vi "closeMightex.vi"   [LabVIEW 2016]
uses:
  lib/SSClassic_USBCamera_SDK.dll
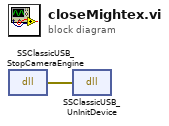
[diagram p0: block diagram]
diagram:
  n1 = dll-call lib="D:/All users/PoSheng/src/lib/SSClassic_USBCamera_SDK.dll" fn="SSClassicUSB_StopCameraEngine" ("CCD_USBCamera_SDK.dll:CCDUSB_StopCameraEngine")() -> (error out=w1:errorcluster)  [unwired: 4 in, 1 out]
  n2 = dll-call lib="D:/All users/PoSheng/src/lib/SSClassic_USBCamera_SDK.dll" fn="SSClassicUSB_UnInitDevice" ("CCD_USBCamera_SDK.dll:CCDUSB_UnInitDevice")(error in=w1) -> ()  [unwired: 3 in, 2 out]
